vi "arctan test.vi"() -> ()   [LabVIEW 2021]
panel:
  out "x/y":dbl
  out "Numeric":dbl
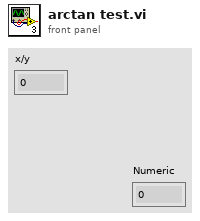
[diagram p1: front panel]
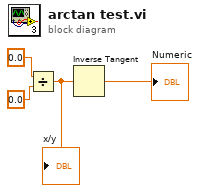
[diagram p0: block diagram]
diagram:
  n1 = Divide(x=0.0, y=0.0 ("x")) -> (x/y=w1:dbl)
  "x/y" <- w1
  n2 = Inverse Tangent(1:w1) -> (0:→"Numeric":dbl)
